vi "FTW-TransferClient-Upload.vi"(0 "Transfer Client":refnum<class "FTW-TransferClient.lvclass">, 5 "Data":string, 7 "Remote Filename":string, 11 "error in":errorcluster) -> (4 "Transfer Client out":refnum<class "FTW-TransferClient.lvclass">, 6 "URI":string, 8 "Response":string, 10 "Upload Time":u32 format="%06dmsec", 15 "error out":errorcluster)   [LabVIEW 2014, in "FTW-TransferClient.lvclass"]
uses:
  FTW-TransferClient.lvclass
panel:
  # "Inputs"
  # "Outputs"
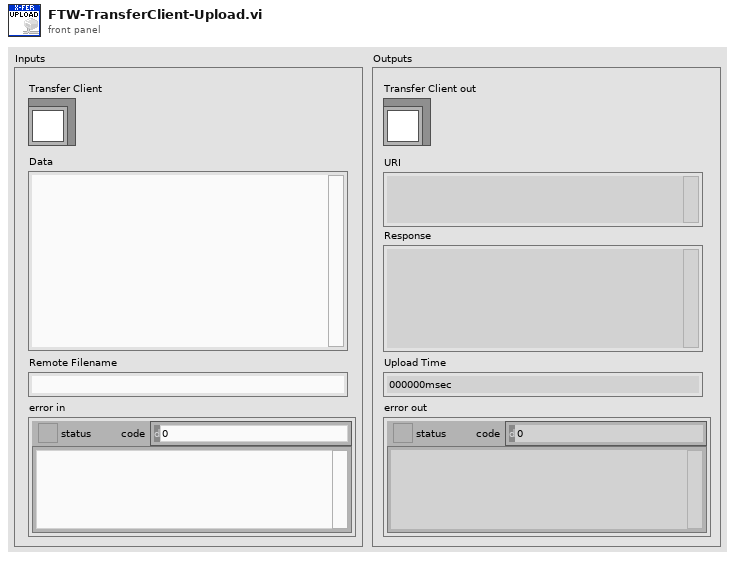
[diagram p1: front panel]
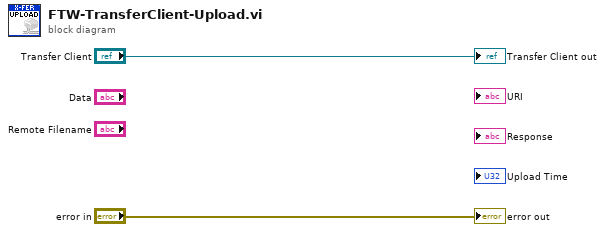
[diagram p0: block diagram]
diagram:
  "error out" <- "error in"
  "Transfer Client out" <- "Transfer Client"
